vi "HGF_Factory.appendData2Variant.vi"(0 "initData":variant, 1 "objectName":string, 5 "error in (no error)":errorcluster, 6 "className":string) -> (14 "dup initData":variant, 19 "error out":errorcluster)   [LabVIEW 2014, in "HGF_BaseClasses.lvlib" / "HGF_Factory.lvclass"]
uses:
  HGF_Factory.lvclass
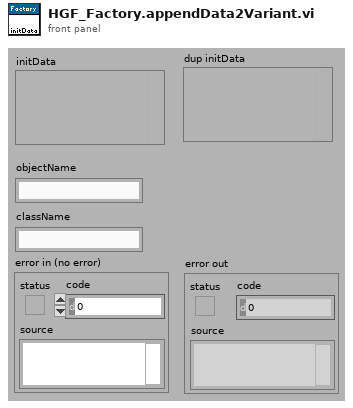
[diagram p1: front panel]
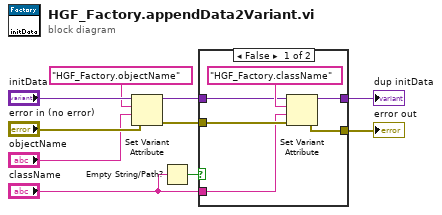
[diagram p0: block diagram]
diagram:
  n1 = Set Variant Attribute(Variant="initData", name="HGF_Factory.objectName", value="objectName", error in="error in (no error)") -> (Variant out=w6:variant, error out=w5:errorcluster)  [unwired: 1 out]
  n2 = Empty String/Path?(string/path="className") -> (empty?=w1:bool)
  n3 = case shown="False" w1 {
    tunnel: w6 -> [w15 w18]
    tunnel: w5 -> [w14 w17]
    tunnel: [w13 w18] -> w4
    tunnel: [w12 w17] -> w3
    tunnel: "className" -> [w11 _]
    frame False {
      n4 = Set Variant Attribute(Variant=w15, name="HGF_Factory.className", value=w11, error in=w14) -> (Variant out=w13:variant, error out=w12:errorcluster)  [unwired: 1 out]
    }
    frame True {
    }
  }
  "dup initData" <- w4
  "error out" <- w3
